vi "Test_MCListboxItemNamesBinding_ValueOK.vi"(8 "error in (no error)":errorcluster, 11 "TestCase in":refnum<class "TestTransport.lvclass">) -> (0 "error out":errorcluster, 3 "TestCase out":refnum<class "TestTransport.lvclass">)   [LabVIEW 2017, in "TestTransport.lvclass"]
uses:
  TestTransport.lvclass
  Source/Framework/Transport/MCListboxItemNamesBinding/MCListboxItemNamesBinding.lvclass/MCListboxItemNamesBinding.ctl
  Source/Framework/Transport/MCListboxItemNamesBinding/MCListboxItemNamesBinding.lvclass
panel:
  out "MCListbox":i32(listbox)
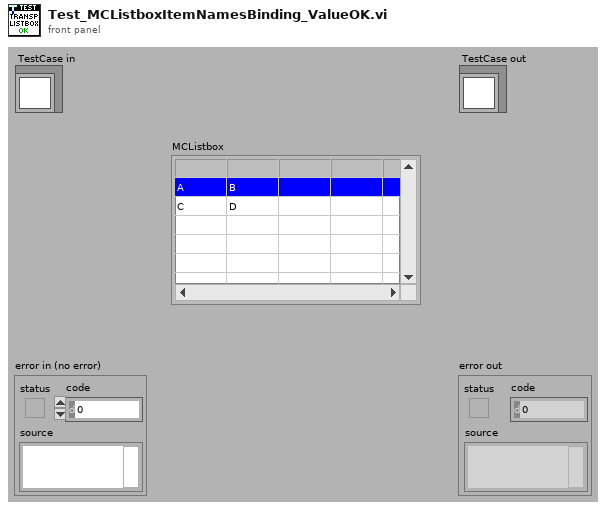
[diagram p1: front panel]
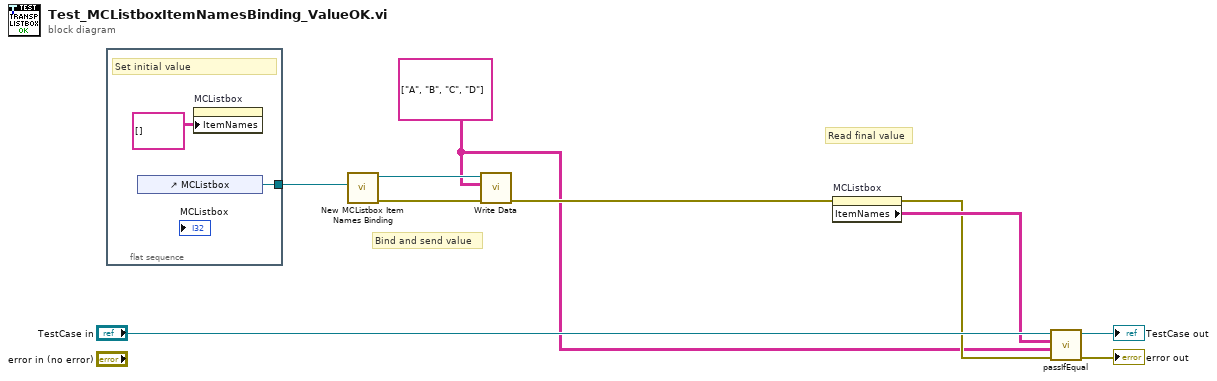
[diagram p0: block diagram]
diagram:
  w2 = string[][] [["A", "B"], ["C", "D"]] ("Item Names")
  # "Bind and send value"
  # "Read final value"
  n1 = flat-sequence {
    tunnel: [w12] -> w1
    frame #0 {
      # "Set initial value"
      n2 = control-ref of="MCListbox"() -> (w12:refnum<vi>)
      n3 = property on="MCListbox" class="MCListbox (strict)"("ItemNames"=string[][] [] ("Item Names")) -> ()  [unwired: 2 in, 2 out]
    }
  }
  n4 = call "New MCListbox Item Names Binding.vi"("MCListbox Refnum"=w1) -> ("error out"=w4:errorcluster, "MCListboxItemNamesBinding"=w6:refnum<class "MCListboxItemNamesBinding.lvclass">)  [unwired: 9 in]
  n5 = call-dynamic "Write Data.vi"("error in (no error)"=w4, "Value"=w2, "MCListboxItemNamesBinding In"=w6) -> ("error out"=w5:errorcluster)  [unwired: 7 in, 1 out]
  n6 = property on="MCListbox" class="MCListbox (strict)"(error in=w5) -> (error out=w3:errorcluster, "ItemNames"=w7:string[][])  [unwired: 1 in, 1 out]
  n7 = call-dynamic "passIfEqual.vi"("error in (no error)"=w3, "y"=w2, "x"=w7, "TestCase in"="TestCase in") -> ("error out"=→"error out":errorcluster, "TestCase out"=→"TestCase out":refnum<class "TestTransport.lvclass">)  [unwired: 6 in]
